vi "Configure Measurement.vi"(6 "Manual Range (1.0)":dbl=1.0 format="%.2f", 7 "Enable Auto Range (True)":bool=TRUE, 8 "error in (no error)":errorcluster, 9 "Resolution (1: 6.5 Digits)":i32(ring)=1 items=["5.5 Digits", "6.5 Digits", "7.5 Digits", "8.5 Digits"], 10 "Function (0: DC Volts)":u16(ring) items=["DC Volts", "AC Volts", "DC Current", "AC Current", "Normal Resistance", "High Voltage Resistance", "True Resistance"], 11 "VISA resource name":refnum<visa-resource-name>) -> (0 "error out":errorcluster, 3 "VISA resource name out":refnum<visa-resource-name>)   [LabVIEW 2012, in "Fluke 8508.lvlib"]
doc: "This VI sets the measurement function on the instruemnt as well as the resolution and range for the particular function.\n\nNOTE: \n(1) For temperature measurements, refer to the temperature subVIs (Configure Temperature and the various conversion VIs).\n(2) For measurement function specific settings use the Configure <measurement function> VIs."
uses:
  Fluke 8508.lvlib
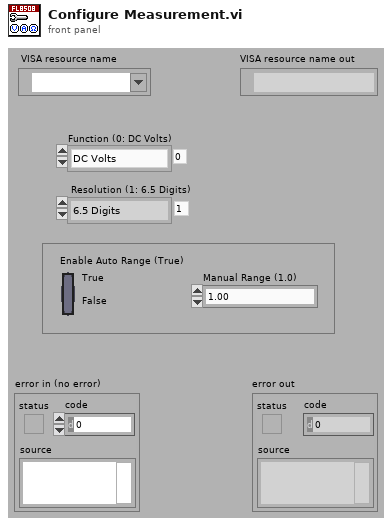
[diagram p1: front panel]
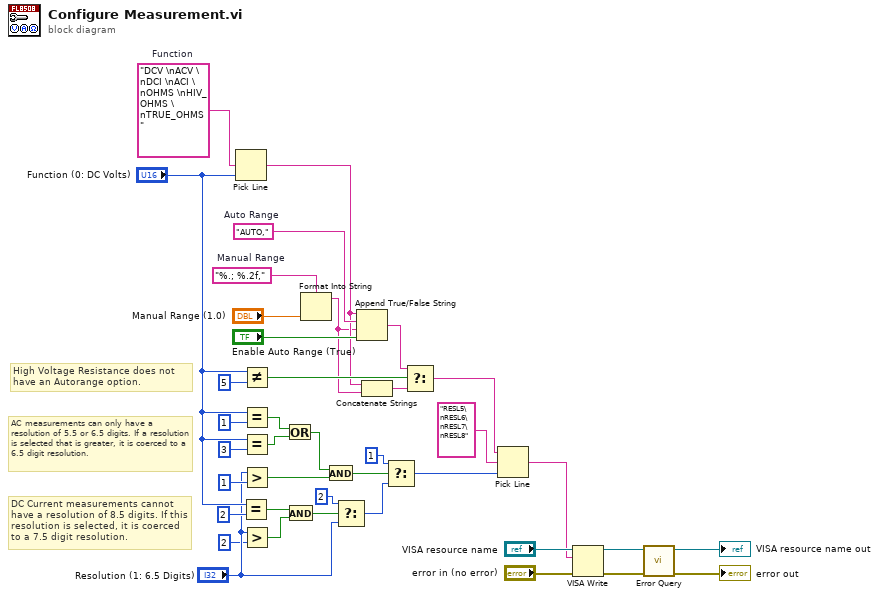
[diagram p0: block diagram]
diagram:
  w32 = "AUTO,"  # Auto Range
  w36 = "%.; %.2f,"  # Manual Range
  w37 = "DCV \nACV \nDCI \nACI \nOHMS \nHIV_OHMS \nTRUE_OHMS "  # Function
  # "DC Current measurements cannot have a resolution of 8.5 digits. If this resolution is selected, it is coerced to a 7.5 digit resolution."
  # "AC measurements can only have a resolution of 5.5 or 6.5 digits. If a resolution is selected that is greater, it is coerced to a 6.5 digit resolution."
  # "High Voltage Resistance does not have an Autorange option."
  n1 = Pick Line(multi-line string=w37, line index="Function (0: DC Volts)") -> (output string=w21:string)  [unwired: 1 in]
  n2 = Equal?(x="Function (0: DC Volts)", y=u16 2) -> (x = y?=w8:bool)
  n3 = Not Equal?(x="Function (0: DC Volts)", y=u16 5) -> (x != y?=w26:bool)
  n4 = Equal?(x="Function (0: DC Volts)", y=u16 1) -> (x = y?=w19:bool)
  n5 = Equal?(x="Function (0: DC Volts)", y=u16 3) -> (x = y?=w15:bool)
  n6 = Greater?(x="Resolution (1: 6.5 Digits)", y=1) -> (0:w11:bool)
  n7 = Greater?(x="Resolution (1: 6.5 Digits)", y=2) -> (0:w2:bool)
  n8 = Or(x=w19, y=w15) -> (x .or. y?=w18:bool)
  n9 = And(x=w8, y=w2) -> (x .and. y?=w6:bool)
  n10 = Format Into String(format string=w36, "Manual Range (1.0)") -> (resulting string=w20:string)  [unwired: 2 in, 1 out]
  n11 = And(x=w18, y=w11) -> (x .and. y?=w17:bool)
  n12 = Select(t=u16 2 ("y"), s=w6, f="Resolution (1: 6.5 Digits)") -> (s? t:f=w1:i32)
  n13 = Append True/False String(1:"Enable Auto Range (True)", 2:w20, 3:w32, 4:w21) -> (0:w24:string)
  n14 = Concatenate Strings(w21, w20) -> (w22:string)
  n15 = Select(t=u16 1 ("y"), s=w17, f=w1) -> (s? t:f=w7:i32)
  n16 = Select(t=w24, s=w26, f=w22) -> (s? t:f=w25:string)
  n17 = Pick Line(string ("")=w25, multi-line string="RESL5\nRESL6\nRESL7\nRESL8", line index=w7) -> (output string=w31:string)
  n18 = VISA Write(VISA resource name="VISA resource name", write buffer=w31, error in (no error)="error in (no error)") -> (VISA resource name out=w29:refnum<visa-resource-name>, error out=w30:errorcluster)  [unwired: 1 out]
  n19 = call "Error Query.vi"("error in (no error)"=w30, "VISA resource name"=w29) -> ("error out"=→"error out":errorcluster, "VISA resource name out"=→"VISA resource name out":refnum<visa-resource-name>)  [unwired: 6 in, 2 out]
